vi "Pasco Auton Pack.vi"(0 "Left Drive":dbl, 1 "Right Drive":dbl, 2 "RAMP ACT":dbl, 3 "Conveyor":dbl, 4 "Harvestor":dbl, 5 "Shooter":dbl, 7 "PIDARRAY":dbl[][](array[numeric]), 9 "Iterations":i32, 11 "Alloted Amount":i32) -> (16 "output array":dbl[][](array[numeric]))   [LabVIEW 2011]
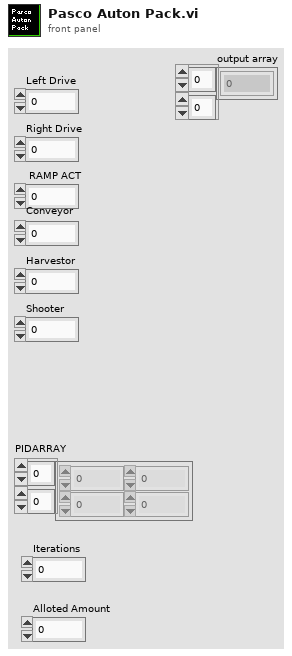
[diagram p1: front panel]
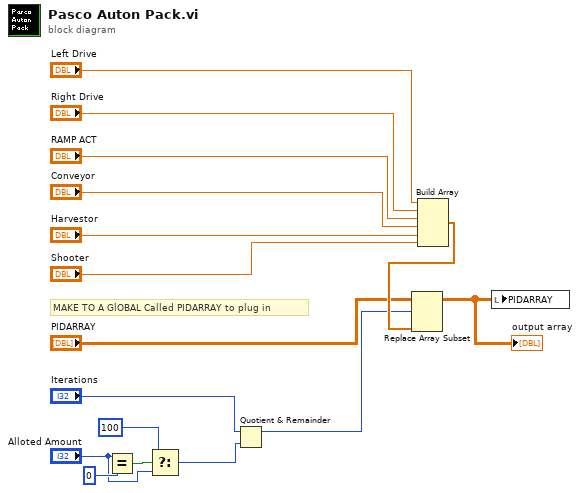
[diagram p0: block diagram]
diagram:
  # "MAKE TO A GlOBAL Called PIDARRAY to plug in"
  n1 = Equal?(x="Alloted Amount", y=0) -> (x = y?=w7:bool)
  n2 = Select(t=100, s=w7, f="Alloted Amount") -> (s? t:f=w3:i32)
  n3 = Quotient & Remainder(x="Iterations", y=w3) -> (x-y*floor(x/y)=w1:i32)  [unwired: 1 out]
  n4 = Build Array("Left Drive", "Right Drive", "RAMP ACT", "Conveyor", "Harvestor", "Shooter") -> (w16:dbl[])
  n5 = Replace Array Subset(array="PIDARRAY", new element=w16, index (row)=w1) -> (w14:dbl[][])  [unwired: 1 in]
  "output array" <- w14
  n6 = local write "PIDARRAY"(w14) -> ()
